vi "LayerGraphicManipulation.vi"(6 "Ref Color":u32(colorbox), 7 "Radio Buttons":T1=enum."Ellipse", 8 "error in":errorcluster, 9 "New Color":u32(colorbox), 10 "point(x,y)":cluster{"x":i16, "y":i16}, 11 "Layer.lvclass":refnum<class "Layer.lvclass">) -> (0 "error out":errorcluster, 2 "Operation processed?":bool, 3 "Layer.lvclass out":refnum<class "Layer.lvclass">)   [LabVIEW 2020, in "Tools Paint.lvclass"]
uses:
  Class/Tools/Tools Paint.lvclass
  vi.lib/LabVIEW Icon API/lv_icon/Classes/Layer/Layer.lvclass
  Class/Tools/Tools Paint.lvclass/Tools Paint.ctl
  vi.lib/LabVIEW Icon API/LabVIEW Icon API.lvlib
  lv_icon.lvlib
  Controls/Circle.ctl
  Controls/Dropper.ctl
  Controls/FCircle.ctl
  Controls/Fill.ctl
  Controls/FRect.ctl
  Controls/Line.ctl
  Controls/Move.ctl
  Controls/Pen.ctl
  Controls/IERect.ctl
  Controls/Rubber.ctl
  Controls/Selection.ctl
  Controls/Text.ctl
  Controls/Tools.ctl
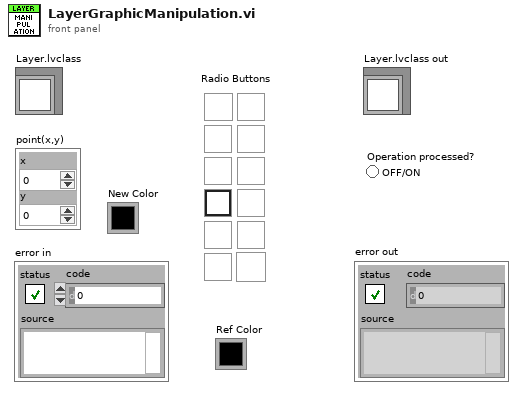
[diagram p1: front panel]
types:
  T1 = typedef "Tools.ctl" = enum32{"Pencil", "Line", "Dropper", "Fill", "Rectangle", "Filled Rectangle", "Ellipse", "Filled Ellipse", "Eraser", "Text", "Select", "Move"}
  T2 = typedef "Layer.ctl" = cluster{"LayerIcon":picture, "LayerName":string, "Opacity":u8, "Visibility?":bool}
  T3 = typedef "LVPoint32TypeDef.ctl" = cluster{"Horizontal":i32, "Vertical":i32}
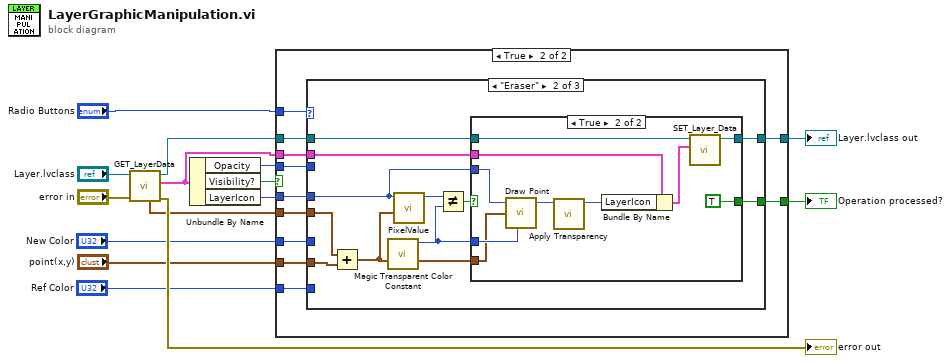
[diagram p0: block diagram]
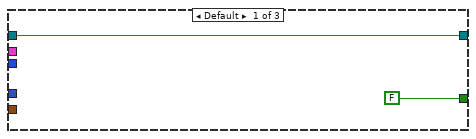
[diagram p3: hidden frame]
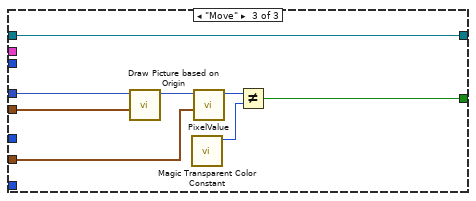
[diagram p5: hidden frame]
diagram:
  n1 = call-dynamic "GET_LayerData.vi"("error in (no error)"="error in", "Layer.lvclass in"="Layer.lvclass") -> ("error out"=→"error out":errorcluster, "Data"=w11:T2, "Layer.lvclass out"=w12:refnum<class "Layer.lvclass">, "Origin"=w9:T3)  [unwired: 6 out]
  n2 = Unbundle By Name(w11) -> ("Opacity"=w6:u8, "Visibility?"=w5:bool, "LayerIcon"=w10:picture)
  n3 = case shown="True" w5 {
    tunnel: w9 -> [_ w26]
    tunnel: w6 -> [_ w20]
    tunnel: w10 -> [_ w27]
    tunnel: "point(x,y)" -> [_ w25]
    tunnel: w11 -> [_ w24]
    tunnel: w12 -> [w16 w23]
    tunnel: [w16 w22] -> w13
    tunnel: "Radio Buttons" -> [_ w21]
    tunnel: [_ w19] -> w3
    tunnel: "New Color" -> [_ w18]
    tunnel: "Ref Color" -> [_ w17]
    frame False {
    }
    frame True {
      n4 = case shown="\"Eraser\"" w21 {
        tunnel: w27 -> [_ w34 w60]
        tunnel: w26 -> [_ w33 w58]
        tunnel: w25 -> [_ w32 w57]
        tunnel: w24 -> [_ w38 _]
        tunnel: w23 -> [w29 w37 w55]
        tunnel: [w29 w36 w55] -> w22
        tunnel: w20 -> [_ _ _]
        tunnel: [FALSE w35 w54] -> w19
        tunnel: w18 -> [_ _ _]
        tunnel: w17 -> [_ _ _]
        frame Default {
        }
        frame "Eraser" {
          n5 = Add(x=w33, y=w32) -> (x+y=w31:T3)
          n6 = call "Magic Transparent Color Constant.vi"() -> ("Magic transparent color constant"=w30:u32)  [unwired: 11 out]
          n7 = call "PixelValue.vi"("point(x,y)"=w31, "Picture"=w34) -> ("Color"=w40:u32)  [unwired: 9 out]
          n8 = Not Equal?(x=w40, y=w30) -> (x != y?=w39:bool)
          n9 = case shown="True" w39 {
            selector: w39 -> [w41 _]
            tunnel: w30 -> [_ w51]
            tunnel: w31 -> [_ w50]
            tunnel: w38 -> [_ w49]
            tunnel: w34 -> [_ w48]
            tunnel: w37 -> [w42 w46]
            tunnel: [w42 w45] -> w36
            tunnel: [w41 TRUE] -> w35
            frame False {
            }
            frame True {
              n10 = call <vilib>:"Draw Point.vi"("picture"=w48, "point(x,y)"=w50, "color(black)"=w51) -> ("new picture"=w52:picture)  [unwired: 1 in, 5 out]
              n11 = call "Apply Transparency.vi"("in"=w52) -> ("out"=w43:picture)  [unwired: 10 in]
              n12 = Bundle By Name(cluster=w49, "LayerIcon"=w43) -> (w47:T2)
              n13 = call-dynamic "SET_Layer_Data.vi"("Data"=w47, "Layer.lvclass in"=w46) -> ("Layer.lvclass out"=w45:refnum<class "Layer.lvclass">)  [unwired: 2 in, 7 out]
            }
          }
        }
        frame "Move" {
          n14 = call "Draw Picture based on Origin.vi"("Origin"=w58, "LayerIcon in"=w60) -> ("LayerIcon out"=w56:picture)  [unwired: 1 in, 8 out]
          n15 = call "Magic Transparent Color Constant.vi"() -> ("Magic transparent color constant"=w53:u32)  [unwired: 11 out]
          n16 = call "PixelValue.vi"("point(x,y)"=w57, "Picture"=w56) -> ("Color"=w59:u32)  [unwired: 9 out]
          n17 = Not Equal?(x=w59, y=w53) -> (x != y?=w54:bool)
        }
      }
    }
  }
  "Layer.lvclass out" <- w13
  "Operation processed?" <- w3
